vi "000 Client Launch.vi"(8 "error in (no error)":errorcluster caption="Error In", 11 "Queue Ref":T1={"UI"=refnum, "Message"=refnum, "Data"=refnum, "Caller"=refnum, "Name"="000 Common", "Data Path"=path "", "Class Path"=path "", "SubPanel"=refnum, "Project Name"="", "MNT"="", "Title"="", "Data Source"=refnum, "Queue List"={}, "VI"=refnum, "UE"=refnum}) -> (0 "error out":errorcluster caption="Error Out")   [LabVIEW 2020]
uses:
  000 Module Data Type.ctl
  Queue Message.ctl
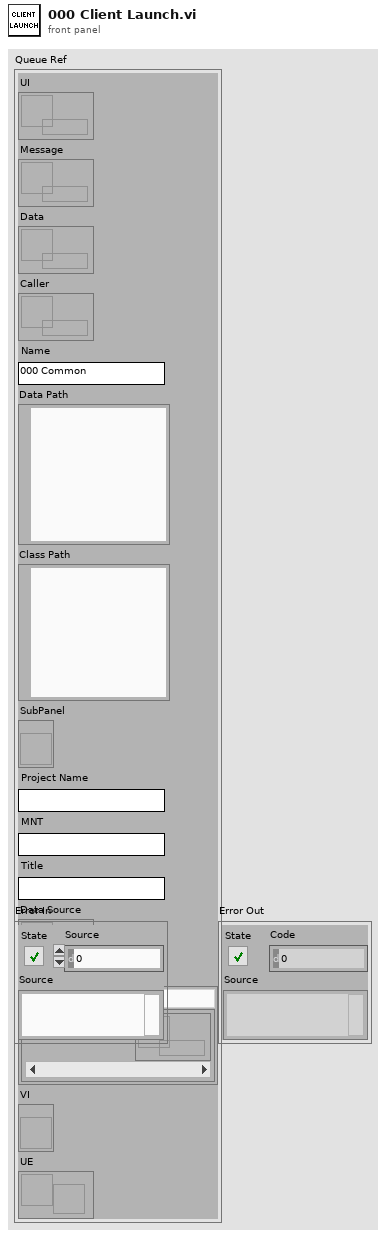
[diagram p1: front panel]
types:
  T1 = typedef "000 Module Data Type.ctl" = cluster{"UI":refnum<queue>, "Message":refnum<queue>, "Data":refnum<queue>, "Caller":refnum<queue>, "Name":string, "Data Path":path, "Class Path":path, "SubPanel":refnum<vi>, "Project Name":string, "MNT":string, "Title":string, "Data Source":refnum<queue>, "Queue List":map{string, refnum<queue>}, "VI":refnum<vi>, "UE":refnum<user-event>}
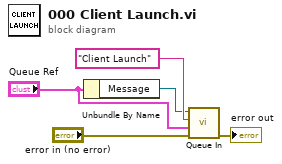
[diagram p0: block diagram]
diagram:
  n1 = Unbundle By Name("Queue Ref") -> ("Message"=w4:refnum<queue>)
  n2 = call "Queue In.vi"("error in (no error)"="error in (no error)", "Data"="Queue Ref", "Message"="Client Launch", "Queue In"=w4) -> ("error out"=→"error out":errorcluster)  [unwired: 6 in, 1 out]
